vi "FileInput.vi"(5 "error in (no error)":errorcluster) -> (14 "Path":path, 19 "error out":errorcluster)   [LabVIEW 2012]
doc: "Displays a standard dialog box that prompts users to enter information, such as a user name and password.\n--------------------\n\nThis Express VI is configured as follows:\n\nMessage to Display to the User:\nThe inputs are: \nText Entry Box: User\nText Entry Box: Path\nText Entry Box: Camera"
panel:
  in  "CSV file Path":path
  in  "Enable":bool=TRUE
  in  "OK":bool caption="OK2"
  out "OK":bool
  # "File & Input Selection"
  # "1. ¶}±ÒÀÉ®× (ÀÉ¦W:XXX.csv)0"
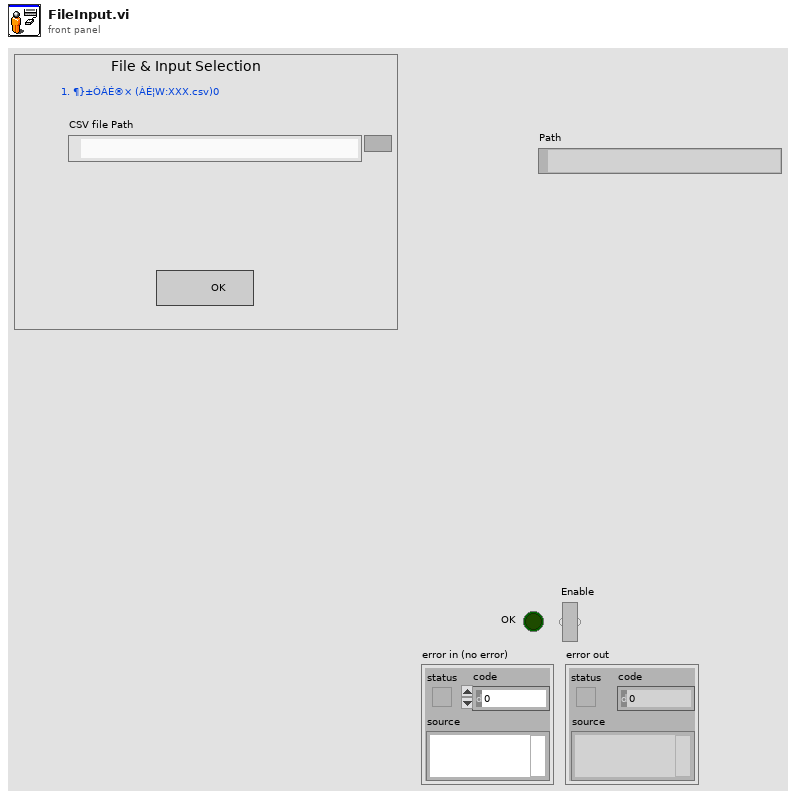
[diagram p1: front panel]
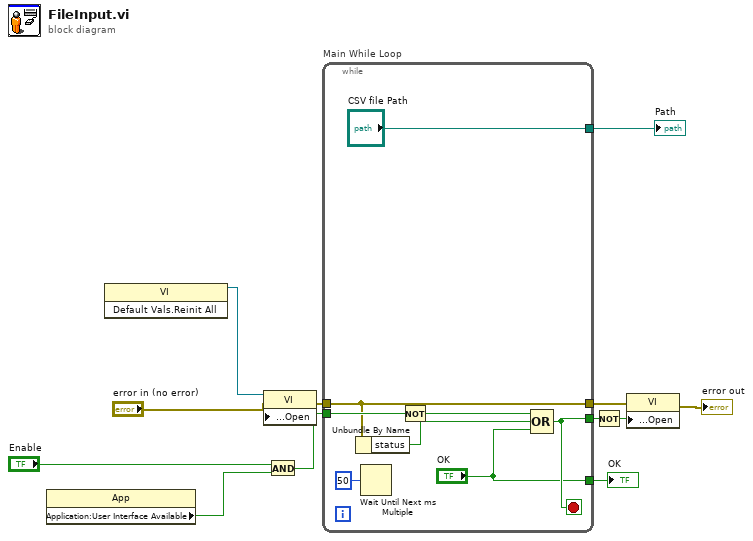
[diagram p0: block diagram]
diagram:
  n1 = property class="App"() -> ("Application:User Interface Available"=w4:bool)  [unwired: 2 in, 2 out]
  n2 = invoke class="VI" method="Default Vals.Reinit All"() -> (reference out=w3:refnum<vi>)  [unwired: 3 in, 2 out]
  n3 = And(x="Enable", y=w4) -> (x .and. y?=w5:bool)
  n4 = property class="VI"(reference=w3, error in="error in (no error)", "Front Panel Window:Open"=w5) -> (error out=w9:errorcluster)  [unwired: 1 out]
  n5 = while "Main While Loop" {
    tunnel: ["OK"] -> w12
    tunnel: w5 -> [w19]
    tunnel: [w17] -> w10
    tunnel: w9 -> [w16]
    tunnel: [w16] -> w8
    tunnel: ["CSV file Path"] -> w2
    stop <- w17 stop-if-true
    n6 = Unbundle By Name(w16) -> ("status"=w15:bool)
    n7 = Wait Until Next ms Multiple(millisecond multiple=u32 50) -> ()  [unwired: 1 out]
    n8 = Not(x=w19) -> (.not. x?=w18:bool)
    n9 = Compound Arithmetic op=OR(w18, w15, "OK") -> (w17:bool)
  }
  "OK" <- w12
  "Path" <- w2
  n10 = Not(x=w10) -> (.not. x?=w11:bool)
  n11 = property class="VI"(error in=w8, "Front Panel Window:Open"=w11) -> (error out=→"error out":errorcluster)  [unwired: 1 in, 1 out]
